vi "VMI_split_data_arrays.vi"(0 "Big_image Array in":i16[][][](array[numeric]), 1 "Peak Array in":cluster{"X":sgl, "Y":sgl}[][](array[cluster]), 2 "Histogram in":i32[][](array[numeric]), 3 "xaxis in":i32[][](array[numeric]), 4 "Powers in":dbl[][](array[numeric]), 5 "Power Err in":dbl[][](array[numeric]), 9 "ArrayIndex":i32) -> (14 "Big_image Array out":i16[][](array[numeric]), 15 "Peak Array out":cluster{"X":sgl, "Y":sgl}[](array[cluster]), 16 "Histogram out":i32[](array[numeric]), 17 "xaxis out":i32[](array[numeric]), 18 "Powers out":dbl[](array[numeric]), 19 "Power Err out":dbl[](array[numeric]))   [LabVIEW 2015]
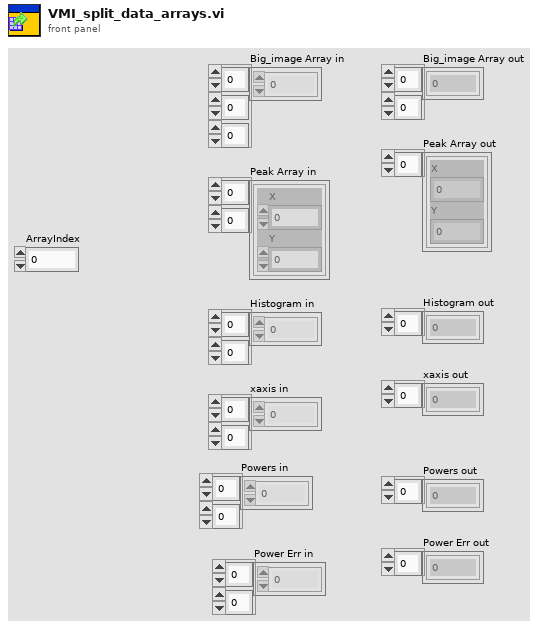
[diagram p1: front panel]
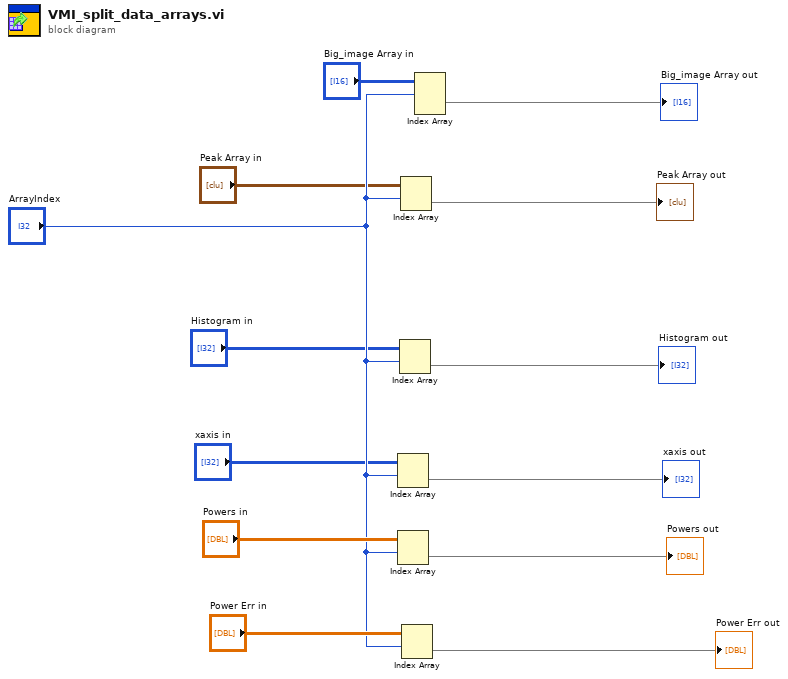
[diagram p0: block diagram]
diagram:
  n1 = Index Array(array="xaxis in", index (row)="ArrayIndex") -> (element=→"xaxis out":i32[])  [unwired: 1 in]
  n2 = Index Array(array="Powers in", index (row)="ArrayIndex") -> (element=→"Powers out":dbl[])  [unwired: 1 in]
  n3 = Index Array(array="Histogram in", index (row)="ArrayIndex") -> (element=→"Histogram out":i32[])  [unwired: 1 in]
  n4 = Index Array(array="Peak Array in", index (row)="ArrayIndex") -> (element=→"Peak Array out":cluster{"X":sgl, "Y":sgl}[])  [unwired: 1 in]
  n5 = Index Array(array="Power Err in", index (row)="ArrayIndex") -> (element=→"Power Err out":dbl[])  [unwired: 1 in]
  n6 = Index Array(array="Big_image Array in", index (dim 0)="ArrayIndex") -> (element=→"Big_image Array out":i16[][])  [unwired: 2 in]
